vi "Create Cube.vi"() -> (3 "Cube":T1)   [LabVIEW 2022 SP3, in "3D.lvlib"]
uses:
  3D.lvlib
  Vector 3D.ctl
  Triangle 3D.ctl
  Object.ctl
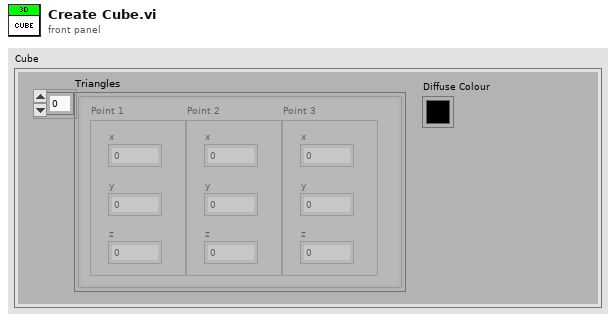
[diagram p1: front panel]
types:
  T1 = typedef "3D.lvlib/Object.ctl" = cluster{"Triangles":T2[], "Diffuse Colour":u32}
  T2 = typedef "3D.lvlib/Triangle 3D.ctl" = cluster{"Point 1":T3, "Point 2":T3, "Point 3":T3}
  T3 = typedef "3D.lvlib/Vector 3D.ctl" = cluster{"x":sgl, "y":sgl, "z":sgl}
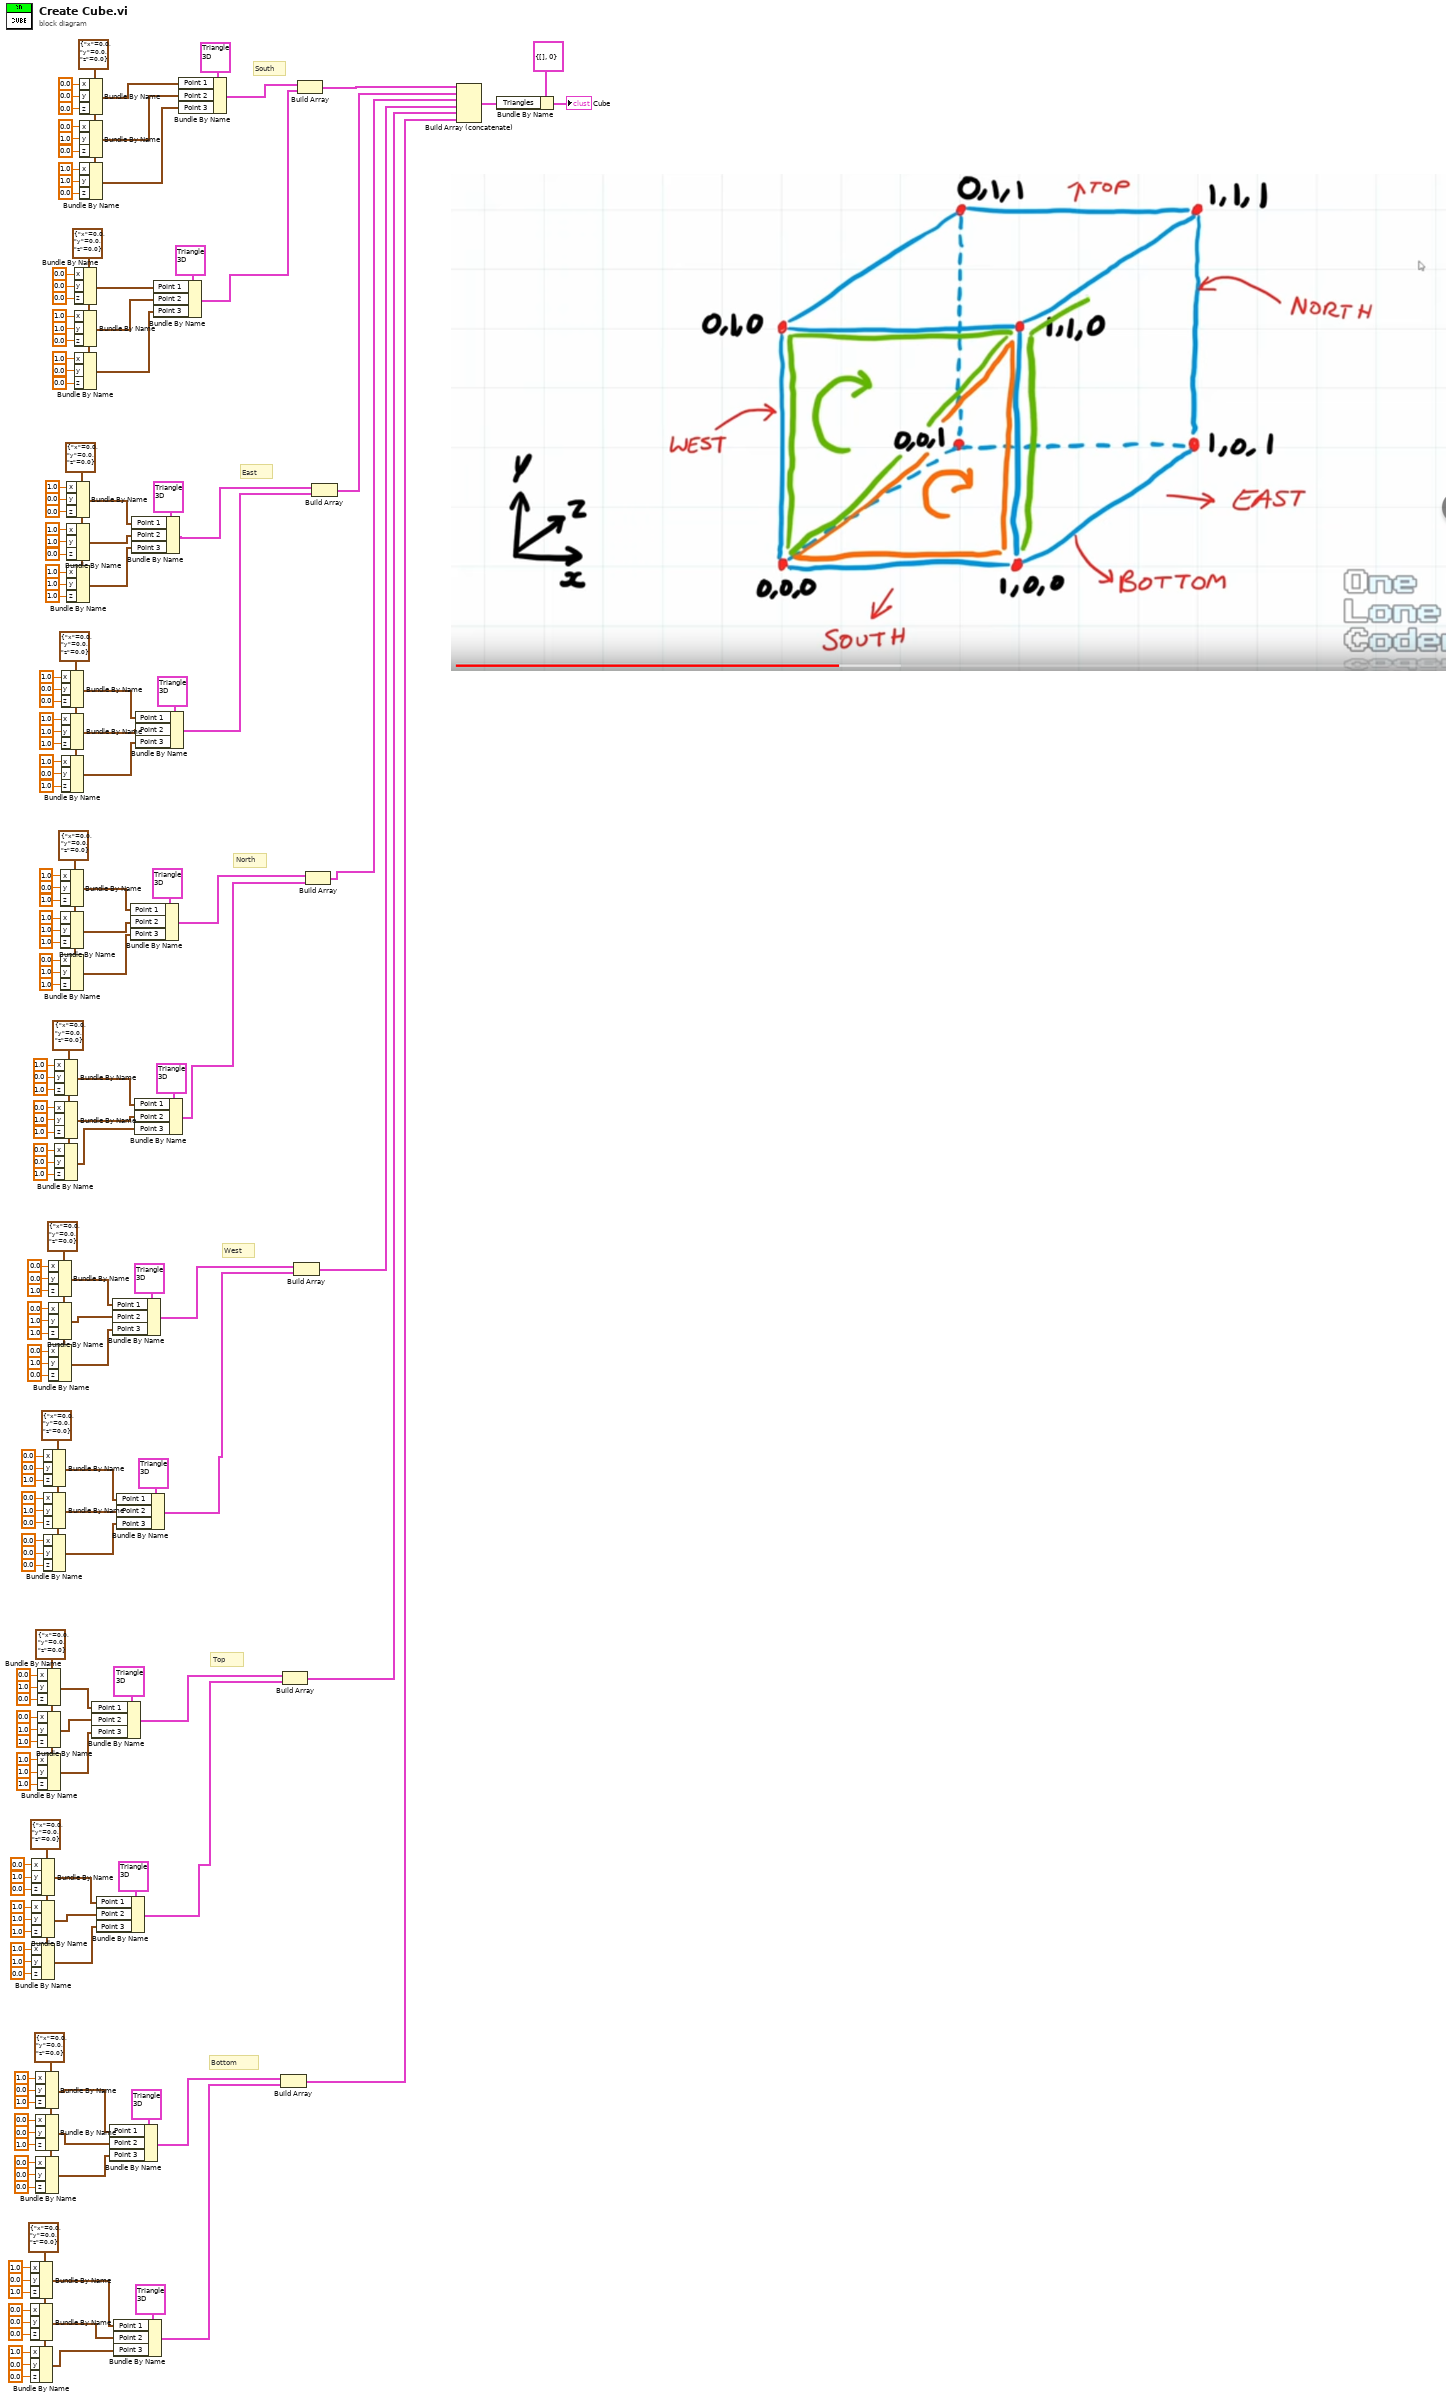
[diagram p0: block diagram]
diagram:
  w76 = T3 {"x"=0.0, "y"=0.0, "z"=0.0} ("Vector 3D")
  w75 = T3 {"x"=0.0, "y"=0.0, "z"=0.0} ("Vector 3D")
  w95 = T3 {"x"=0.0, "y"=0.0, "z"=0.0} ("Vector 3D")
  w96 = T3 {"x"=0.0, "y"=0.0, "z"=0.0} ("Vector 3D")
  w116 = T3 {"x"=0.0, "y"=0.0, "z"=0.0} ("Vector 3D")
  w115 = T3 {"x"=0.0, "y"=0.0, "z"=0.0} ("Vector 3D")
  w135 = T3 {"x"=0.0, "y"=0.0, "z"=0.0} ("Vector 3D")
  w136 = T3 {"x"=0.0, "y"=0.0, "z"=0.0} ("Vector 3D")
  w156 = T3 {"x"=0.0, "y"=0.0, "z"=0.0} ("Vector 3D")
  w155 = T3 {"x"=0.0, "y"=0.0, "z"=0.0} ("Vector 3D")
  w175 = T3 {"x"=0.0, "y"=0.0, "z"=0.0} ("Vector 3D")
  w176 = T3 {"x"=0.0, "y"=0.0, "z"=0.0} ("Vector 3D")
  # "Bottom"
  # "Top"
  # "West"
  # "North"
  # "East"
  # "South"
  n1 = Bundle By Name(cluster=w76, "x"=sgl 1.0, "y"=sgl 0.0, "z"=sgl 1.0) -> (w5:T3)
  n2 = Bundle By Name(cluster=w76, "x"=sgl 0.0, "y"=sgl 0.0, "z"=sgl 0.0) -> (w4:T3)
  n3 = Bundle By Name(cluster=w76, "x"=sgl 1.0, "y"=sgl 0.0, "z"=sgl 0.0) -> (w3:T3)
  n4 = Bundle By Name(cluster=w95, "x"=sgl 0.0, "y"=sgl 1.0, "z"=sgl 0.0) -> (w15:T3)
  n5 = Bundle By Name(cluster=w95, "x"=sgl 1.0, "y"=sgl 1.0, "z"=sgl 1.0) -> (w14:T3)
  n6 = Bundle By Name(cluster=w95, "x"=sgl 1.0, "y"=sgl 1.0, "z"=sgl 0.0) -> (w13:T3)
  n7 = Bundle By Name(cluster=w75, "x"=sgl 1.0, "y"=sgl 0.0, "z"=sgl 1.0) -> (w8:T3)
  n8 = Bundle By Name(cluster=w75, "x"=sgl 0.0, "y"=sgl 0.0, "z"=sgl 1.0) -> (w7:T3)
  n9 = Bundle By Name(cluster=w75, "x"=sgl 0.0, "y"=sgl 0.0, "z"=sgl 0.0) -> (w6:T3)
  n10 = Bundle By Name(cluster=w96, "x"=sgl 0.0, "y"=sgl 1.0, "z"=sgl 0.0) -> (w18:T3)
  n11 = Bundle By Name(cluster=w96, "x"=sgl 0.0, "y"=sgl 1.0, "z"=sgl 1.0) -> (w17:T3)
  n12 = Bundle By Name(cluster=w96, "x"=sgl 1.0, "y"=sgl 1.0, "z"=sgl 1.0) -> (w16:T3)
  n13 = Bundle By Name(cluster=w116, "x"=sgl 0.0, "y"=sgl 0.0, "z"=sgl 1.0) -> (w24:T3)
  n14 = Bundle By Name(cluster=w116, "x"=sgl 0.0, "y"=sgl 1.0, "z"=sgl 0.0) -> (w23:T3)
  n15 = Bundle By Name(cluster=w116, "x"=sgl 0.0, "y"=sgl 0.0, "z"=sgl 0.0) -> (w22:T3)
  n16 = Bundle By Name(cluster=w115, "x"=sgl 0.0, "y"=sgl 0.0, "z"=sgl 1.0) -> (w28:T3)
  n17 = Bundle By Name(cluster=w115, "x"=sgl 0.0, "y"=sgl 1.0, "z"=sgl 1.0) -> (w27:T3)
  n18 = Bundle By Name(cluster=w115, "x"=sgl 0.0, "y"=sgl 1.0, "z"=sgl 0.0) -> (w26:T3)
  n19 = Bundle By Name(cluster=w135, "x"=sgl 1.0, "y"=sgl 0.0, "z"=sgl 1.0) -> (w35:T3)
  n20 = Bundle By Name(cluster=w135, "x"=sgl 0.0, "y"=sgl 1.0, "z"=sgl 1.0) -> (w34:T3)
  n21 = Bundle By Name(cluster=w135, "x"=sgl 0.0, "y"=sgl 0.0, "z"=sgl 1.0) -> (w33:T3)
  n22 = Bundle By Name(cluster=w136, "x"=sgl 1.0, "y"=sgl 0.0, "z"=sgl 1.0) -> (w38:T3)
  n23 = Bundle By Name(cluster=w136, "x"=sgl 1.0, "y"=sgl 1.0, "z"=sgl 1.0) -> (w37:T3)
  n24 = Bundle By Name(cluster=w136, "x"=sgl 0.0, "y"=sgl 1.0, "z"=sgl 1.0) -> (w36:T3)
  n25 = Bundle By Name(cluster=w156, "x"=sgl 1.0, "y"=sgl 0.0, "z"=sgl 0.0) -> (w44:T3)
  n26 = Bundle By Name(cluster=w156, "x"=sgl 1.0, "y"=sgl 1.0, "z"=sgl 1.0) -> (w43:T3)
  n27 = Bundle By Name(cluster=w156, "x"=sgl 1.0, "y"=sgl 0.0, "z"=sgl 1.0) -> (w42:T3)
  n28 = Bundle By Name(cluster=w155, "x"=sgl 1.0, "y"=sgl 0.0, "z"=sgl 0.0) -> (w49:T3)
  n29 = Bundle By Name(cluster=w155, "x"=sgl 1.0, "y"=sgl 1.0, "z"=sgl 0.0) -> (w48:T3)
  n30 = Bundle By Name(cluster=w155, "x"=sgl 1.0, "y"=sgl 1.0, "z"=sgl 1.0) -> (w47:T3)
  n31 = Bundle By Name(cluster=w175, "x"=sgl 0.0, "y"=sgl 0.0, "z"=sgl 0.0) -> (w54:T3)
  n32 = Bundle By Name(cluster=w175, "x"=sgl 1.0, "y"=sgl 1.0, "z"=sgl 0.0) -> (w53:T3)
  n33 = Bundle By Name(cluster=w175, "x"=sgl 1.0, "y"=sgl 0.0, "z"=sgl 0.0) -> (w52:T3)
  n34 = Bundle By Name(cluster=w176, "x"=sgl 0.0, "y"=sgl 0.0, "z"=sgl 0.0) -> (w58:T3)
  n35 = Bundle By Name(cluster=w176, "x"=sgl 0.0, "y"=sgl 1.0, "z"=sgl 0.0) -> (w57:T3)
  n36 = Bundle By Name(cluster=w176, "x"=sgl 1.0, "y"=sgl 1.0, "z"=sgl 0.0) -> (w56:T3)
  n37 = Bundle By Name(cluster=T2 {"Point 1"={"x"=0.0, "y"=0.0, "z"=0.0}, "Point 2"={"x"=0.0, "y"=0.0, "z"=0.0}, "Point 3"={"x"=0.0, "y"=0.0, "z"=0.0}} ("Triangle"), "Point 1"=w18, "Point 2"=w17, "Point 3"=w16) -> (w12:T2)
  n38 = Bundle By Name(cluster=T2 {"Point 1"={"x"=0.0, "y"=0.0, "z"=0.0}, "Point 2"={"x"=0.0, "y"=0.0, "z"=0.0}, "Point 3"={"x"=0.0, "y"=0.0, "z"=0.0}} ("Triangle"), "Point 1"=w15, "Point 2"=w14, "Point 3"=w13) -> (w11:T2)
  n39 = Bundle By Name(cluster=T2 {"Point 1"={"x"=0.0, "y"=0.0, "z"=0.0}, "Point 2"={"x"=0.0, "y"=0.0, "z"=0.0}, "Point 3"={"x"=0.0, "y"=0.0, "z"=0.0}} ("Triangle"), "Point 1"=w8, "Point 2"=w7, "Point 3"=w6) -> (w2:T2)
  n40 = Bundle By Name(cluster=T2 {"Point 1"={"x"=0.0, "y"=0.0, "z"=0.0}, "Point 2"={"x"=0.0, "y"=0.0, "z"=0.0}, "Point 3"={"x"=0.0, "y"=0.0, "z"=0.0}} ("Triangle"), "Point 1"=w28, "Point 2"=w27, "Point 3"=w26) -> (w25:T2)
  n41 = Bundle By Name(cluster=T2 {"Point 1"={"x"=0.0, "y"=0.0, "z"=0.0}, "Point 2"={"x"=0.0, "y"=0.0, "z"=0.0}, "Point 3"={"x"=0.0, "y"=0.0, "z"=0.0}} ("Triangle"), "Point 1"=w5, "Point 2"=w4, "Point 3"=w3) -> (w1:T2)
  n42 = Bundle By Name(cluster=T2 {"Point 1"={"x"=0.0, "y"=0.0, "z"=0.0}, "Point 2"={"x"=0.0, "y"=0.0, "z"=0.0}, "Point 3"={"x"=0.0, "y"=0.0, "z"=0.0}} ("Triangle"), "Point 1"=w24, "Point 2"=w23, "Point 3"=w22) -> (w21:T2)
  n43 = Bundle By Name(cluster=T2 {"Point 1"={"x"=0.0, "y"=0.0, "z"=0.0}, "Point 2"={"x"=0.0, "y"=0.0, "z"=0.0}, "Point 3"={"x"=0.0, "y"=0.0, "z"=0.0}} ("Triangle"), "Point 1"=w38, "Point 2"=w37, "Point 3"=w36) -> (w32:T2)
  n44 = Bundle By Name(cluster=T2 {"Point 1"={"x"=0.0, "y"=0.0, "z"=0.0}, "Point 2"={"x"=0.0, "y"=0.0, "z"=0.0}, "Point 3"={"x"=0.0, "y"=0.0, "z"=0.0}} ("Triangle"), "Point 1"=w49, "Point 2"=w48, "Point 3"=w47) -> (w46:T2)
  n45 = Bundle By Name(cluster=T2 {"Point 1"={"x"=0.0, "y"=0.0, "z"=0.0}, "Point 2"={"x"=0.0, "y"=0.0, "z"=0.0}, "Point 3"={"x"=0.0, "y"=0.0, "z"=0.0}} ("Triangle"), "Point 1"=w35, "Point 2"=w34, "Point 3"=w33) -> (w31:T2)
  n46 = Bundle By Name(cluster=T2 {"Point 1"={"x"=0.0, "y"=0.0, "z"=0.0}, "Point 2"={"x"=0.0, "y"=0.0, "z"=0.0}, "Point 3"={"x"=0.0, "y"=0.0, "z"=0.0}} ("Triangle"), "Point 1"=w44, "Point 2"=w43, "Point 3"=w42) -> (w41:T2)
  n47 = Bundle By Name(cluster=T2 {"Point 1"={"x"=0.0, "y"=0.0, "z"=0.0}, "Point 2"={"x"=0.0, "y"=0.0, "z"=0.0}, "Point 3"={"x"=0.0, "y"=0.0, "z"=0.0}} ("Triangle"), "Point 1"=w54, "Point 2"=w53, "Point 3"=w52) -> (w51:T2)
  n48 = Bundle By Name(cluster=T2 {"Point 1"={"x"=0.0, "y"=0.0, "z"=0.0}, "Point 2"={"x"=0.0, "y"=0.0, "z"=0.0}, "Point 3"={"x"=0.0, "y"=0.0, "z"=0.0}} ("Triangle"), "Point 1"=w58, "Point 2"=w57, "Point 3"=w56) -> (w187:T2)
  n49 = Build Array(w2, w1) -> (w61:T2[])
  n50 = Build Array(w12, w11) -> (w62:T2[])
  n51 = Build Array(w25, w21) -> (w63:T2[])
  n52 = Build Array(w187, w51) -> (w60:T2[])
  n53 = Build Array(w32, w31) -> (w64:T2[])
  n54 = Build Array(w46, w41) -> (w65:T2[])
  n55 = Build Array (concatenate)(w60, w65, w64, w63, w62, w61) -> (w59:T2[])
  n56 = Bundle By Name(cluster=T1 {"Triangles"=[], "Diffuse Colour"=0} ("Mesh"), "Triangles"=w59) -> (→"Cube":T1)
